vi "Scale.vi"(1 "Numeric 2":dbl, 2 "Numeric":dbl, 3 "Numeric 3":i32) -> (0 "Cluster":cluster{"Numeric 2":dbl, dbl})   [LabVIEW 2016]
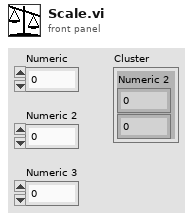
[diagram p1: front panel]
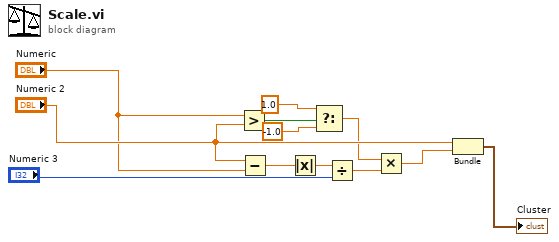
[diagram p0: block diagram]
diagram:
  n1 = Greater?(x="Numeric", y="Numeric 2") -> (0:w2:bool)
  n2 = Subtract(x="Numeric 2", y="Numeric") -> (x-y=w1:dbl)
  n3 = Absolute Value(x=w1) -> (abs(x)=w7:dbl)
  n4 = Select(t=1.0, s=w2, f=-1.0) -> (s? t:f=w5:dbl)
  n5 = Divide(x=w7, y="Numeric 3") -> (x/y=w9:dbl)
  n6 = Multiply(x=w5, y=w9) -> (x*y=w6:dbl)
  n7 = Bundle("Numeric 2"="Numeric 2", w6) -> (→"Cluster":cluster{"Numeric 2":dbl, dbl})  [unwired: 1 in]
